vi "File Write Line.vi"(6 "TD1 Pressure":dbl, 8 "TC Temp":dbl, 9 "TD0 Pressure":dbl, 10 "Timestamp":u32, 11 "file in":refnum<file>) -> (3 "Byte Stream File out":refnum<file>)   [LabVIEW 2015]
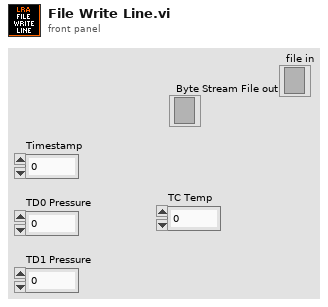
[diagram p1: front panel]
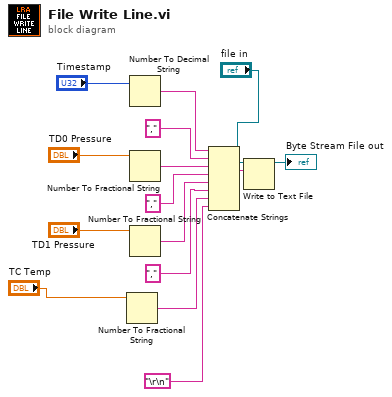
[diagram p0: block diagram]
diagram:
  n1 = Number To Fractional String(number="TC Temp") -> (F-format string=w2:string)  [unwired: 3 in]
  n2 = Number To Decimal String(number="Timestamp") -> (decimal integer string=w9:string)  [unwired: 1 in]
  n3 = Number To Fractional String(number="TD0 Pressure") -> (F-format string=w11:string)  [unwired: 3 in]
  n4 = Number To Fractional String(number="TD1 Pressure") -> (F-format string=w13:string)  [unwired: 3 in]
  n5 = Concatenate Strings(w9, ",", w11, ",", w13, ",", w2, "\r\n") -> (w14:string)
  n6 = Write to Text File(file (use dialog)="file in", text=w14) -> (refnum out=→"Byte Stream File out":refnum<file>)  [unwired: 2 in, 2 out]
